vi "DistanceEstimatorTest.vi"() -> ()   [LabVIEW 2017]
panel:
  out "dist":dbl
  in  "cang":dbl
  in  "ty":dbl
  in  "theight":dbl
  in  "cheight":dbl
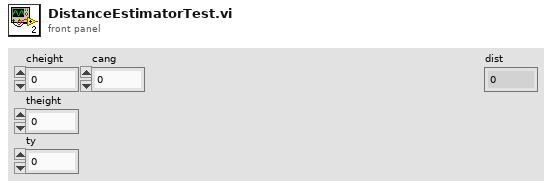
[diagram p1: front panel]
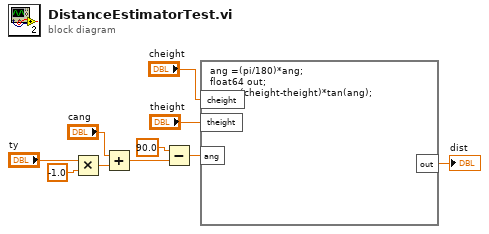
[diagram p0: block diagram]
diagram:
  n1 = Multiply(x="ty", y=-1.0) -> (x*y=w9:dbl)
  n2 = Add(x="cang", y=w9) -> (x+y=w8:dbl)
  n3 = Subtract(x=90.0, y=w8) -> (x-y=w5:dbl)
  n4 = formula code="ang =(pi/180)*ang;\nfloat64 out;\nout = (cheight-theight)*tan(ang);"("cheight"="cheight", "theight"="theight", "ang"=w5) -> ("out"=→"dist":dbl)
